vi "Configure Measurement.vi"(8 "error in (no error)":errorcluster, 9 "Channel Name":string, 10 "measurement configuration":T1={"Pin Name"="", "Time Per Record"=0.0, "Minimum Record Length"=0, "Trigger Level"=0.0, "Vertical Range"=0.0, "Vertical Offset"=10.0, "Probe Attenuation"=1.0, "Vertical Coupling"=1} {"Vertical Coupling" items=["AC", "DC", "GND"]}, 11 "IVI Refnum in":refnum<k15>) -> (0 "error out":errorcluster, 3 "IVI Refnum out":refnum<k15>)   [LabVIEW 2020, in "IVI Scope Measurement.lvlib"]
uses:
  IVI Scope Measurement.lvlib
  Measurement Configuration.ctl
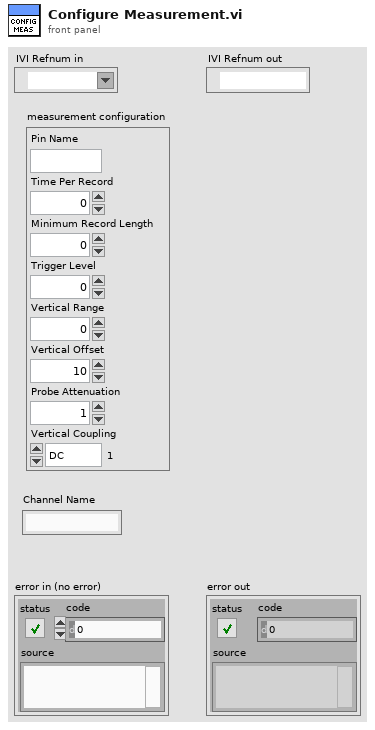
[diagram p1: front panel]
types:
  T1 = typedef "IVI Scope Measurement.lvlib/Measurement Configuration.ctl" = cluster{"Pin Name":string, "Time Per Record":dbl, "Minimum Record Length":i32, "Trigger Level":dbl, "Vertical Range":dbl, "Vertical Offset":dbl, "Probe Attenuation":dbl, "Vertical Coupling":u32}
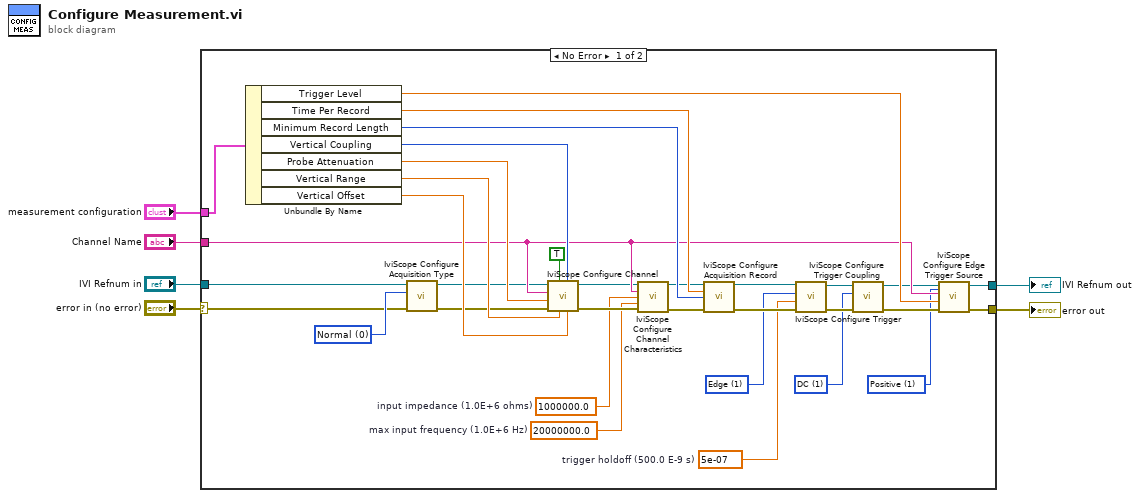
[diagram p0: block diagram]
diagram:
  n1 = case shown="No Error" "error in (no error)" {
    selector: "error in (no error)" -> [w7 w41]
    tunnel: "IVI Refnum in" -> [w39 w40]
    tunnel: [w38 w40] -> w5
    tunnel: [w37 w41] -> w4
    tunnel: "measurement configuration" -> [w36 _]
    tunnel: "Channel Name" -> [w28 _]
    frame No Error {
      w8 = 1 items=["Positive"=1, "Negative"=0] ("trigger slope (Positive)")
      w9 = 1 items=["AC"=0, "DC"=1, "HF Reject"=3, "LF Reject"=4, "Noise Reject"=5] ("trigger coupling (DC)")
      w10 = 5e-07  # trigger holdoff (500.0 E-9 s)
      w11 = 1 items=["Edge"=1, "TV"=5, "Runt"=3, "Glitch"=4, "Width"=2, "AC Line"=7, "Immediate"=6] ("trigger type (Edge)")
      w12 = 20000000.0  # max input frequency (1.0E+6 Hz)
      w13 = 1000000.0  # input impedance (1.0E+6 ohms)
      w16 = 0 items=["Normal", "Peak Detect", "High Resolution", "Envelope", "Average"] ("acquisition type (Normal)")
      n2 = Unbundle By Name(w36) -> ("Trigger Level"=w29:dbl, "Time Per Record"=w33:dbl, "Minimum Record Length"=w34:i32, "Vertical Coupling"=w35:u32, "Probe Attenuation"=w32:dbl, "Vertical Range"=w31:dbl, "Vertical Offset"=w30:dbl)
      n3 = call <vilib>:"IviScope Configure Acquisition Type.vi"("error in (no error)"=w7, "acquisition type (Normal)"=w16, "instrument handle"=w39) -> ("error out"=w17:errorcluster, "instrument handle out"=w19:refnum<k15>)  [unwired: 7 out]
      n4 = call <vilib>:"IviScope Configure Channel.vi"("vertical offset (0.0 V)"=w30, "vertical coupling (DC)"=w35, "vertical range (10.0 V)"=w31, "channel enabled (True)"=TRUE, "error in (no error)"=w17, "probe attenuation (1:1.0)"=w32, "channel name (\"CHANNEL1\")"=w28, "instrument handle"=w19) -> ("error out"=w18:errorcluster, "instrument handle out"=w14:refnum<k15>)  [unwired: 2 out]
      n5 = call <vilib>:"IviScope Configure Channel Characteristics.vi"("instrument handle"=w14, "channel name (\"CHANNEL1\")"=w28, "input impedance (1.0E+6 ohms)"=w13, "max input frequency (1.0E+6 Hz)"=w12, "error in (no error)"=w18) -> ("instrument handle out"=w20:refnum<k15>, "error out"=w21:errorcluster)  [unwired: 9 out]
      n6 = call <vilib>:"IviScope Configure Acquisition Record.vi"("instrument handle"=w20, "time per record (1.0E-3 s)"=w33, "min record length (100 samples)"=w34, "error in (no error)"=w21) -> ("instrument handle out"=w22:refnum<k15>, "error out"=w23:errorcluster)  [unwired: 1 in, 9 out]
      n7 = call <vilib>:"IviScope Configure Trigger.vi"("error in (no error)"=w23, "trigger holdoff (500.0 E-9 s)"=w10, "trigger type (Edge)"=w11, "instrument handle"=w22) -> ("error out"=w25:errorcluster, "instrument handle out"=w24:refnum<k15>)  [unwired: 2 in, 4 out]
      n8 = call <vilib>:"IviScope Configure Trigger Coupling.vi"("error in (no error)"=w25, "trigger coupling (DC)"=w9, "instrument handle"=w24) -> ("error out"=w26:errorcluster, "instrument handle out"=w27:refnum<k15>)  [unwired: 7 out]
      n9 = call <vilib>:"IviScope Configure Edge Trigger Source.vi"("trigger slope (Positive)"=w8, "error in (no error)"=w26, "trigger level  (0.0 V)"=w29, "trigger source (CHANNEL1)"=w28, "instrument handle"=w27) -> ("error out"=w37:errorcluster, "instrument handle out"=w38:refnum<k15>)  [unwired: 1 in, 4 out]
    }
    frame Error {
    }
  }
  "error out" <- w4
  "IVI Refnum out" <- w5
